vi "Add.vi"(8 "error in (no error)":errorcluster, 11 "Module ID":i32=-1) -> (0 "error out":errorcluster, 2 "replaced?":bool, 3 "First?":bool)   [LabVIEW 2019, in "Multiple_uC.lvlib" / "Clone Registration.lvlib"]
doc: "Add a new cloneable module instance ID to the registry.\n_____\nBased on Delacor QMH Project Template 5.0.0.82."
uses:
  Clone Registration.lvlib
  Action--enum.ctl
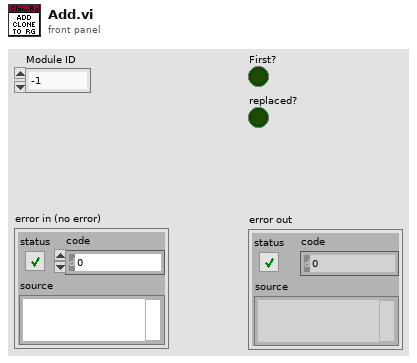
[diagram p1: front panel]
types:
  T1 = typedef "Multiple_uC.lvlib/Clone Registration.lvlib/Action--enum.ctl" = enum16{"Init", "Add Instance", "Remove Instance", "List Instances", "Is First?"}
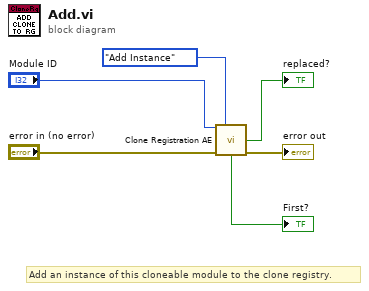
[diagram p0: block diagram]
diagram:
  # "Add an instance of this cloneable module to the clone registry."
  n1 = call "Clone Registration AE.vi"("Module ID"="Module ID", "Action"=Action--enum."Add Instance", "error in"="error in (no error)") -> ("replaced"=→"replaced?":bool, "First?"=→"First?":bool, "error out"=→"error out":errorcluster)  [unwired: 4 in, 6 out]
